vi "Winkel1.vi"() -> ()   [LabVIEW 2013]
panel:
  out "Signalverlaufsdiagramm 2":dbl(graph)
  out "Drehspulinstrument":dbl(knob) scale=175.0..185.0
  out "Rundinstrument":dbl(knob) scale=0.0..360.0 scale format="%#_5g"
  out "Signalverlaufsdiagramm":dbl(graph)
  out "Winkelgeschwindigkeit":dbl format="%#.6f"
  out "Winkel":dbl format="%0.2f"
  in  "Stopp":bool
  in  "z index value":dbl=2.3 caption="z-Index - Wert"
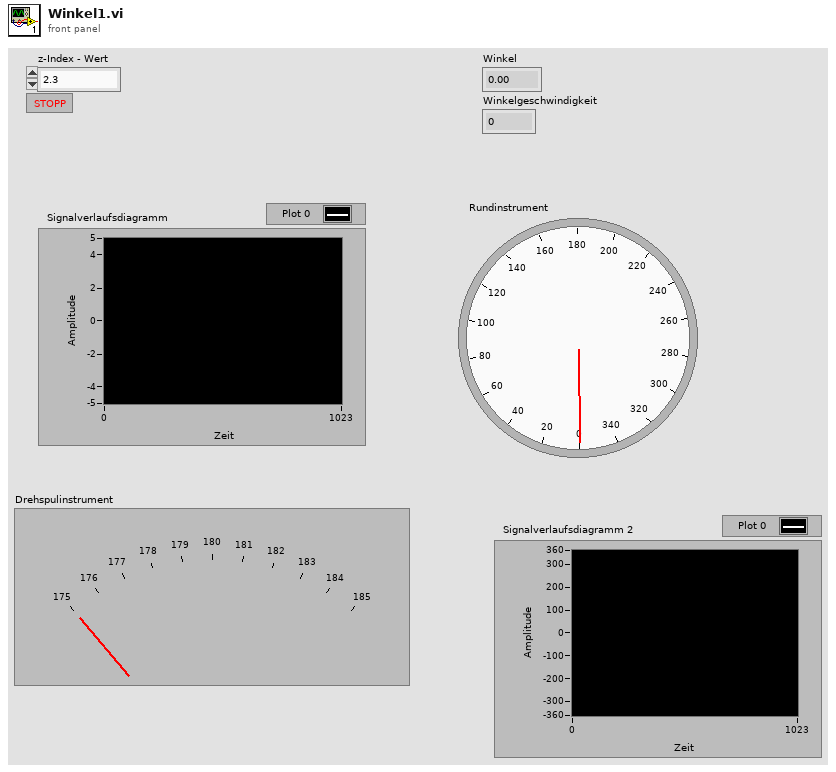
[diagram p1: front panel]
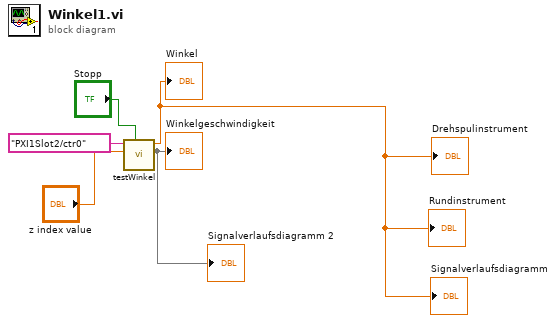
[diagram p0: block diagram]
diagram:
  n1 = call "testWinkel.vi"("Stopp"="Stopp", 10:"z index value", 11:tag "PXI1Slot2/ctr0" ("counter")) -> (2:→"Winkelgeschwindigkeit" →"Signalverlaufsdiagramm 2", "Winkel"=→"Winkel" →"Signalverlaufsdiagramm" →"Rundinstrument" →"Drehspulinstrument":dbl)  [unwired: 7 in]
